vi "Menu Button - Update To Active Level.vi"(7 "RadioButtonsControl in":refnum<vi>, 11 "Display State In in":T1={"Header"="", "Label[]"=[], "DisableButtonsLUT"=variant(string[] []), "Menu Config"=variant}) -> (3 "Display State In out":T1={"Header"="", "Label[]"=[], "DisableButtonsLUT"=variant(string[] []), "Menu Config"=variant})   [LabVIEW 2019, in "Menu Button.xctl"]
doc: "JSMA Module Template - Top Level UI 0.2.0.4\nRob Humfeld - Jet Engineering\nCopyright (c) 2019, Jet Engineering"
uses:
  Menu Button.xctl
  State 1.ctl
  Button Config Cluster STYP.ctl
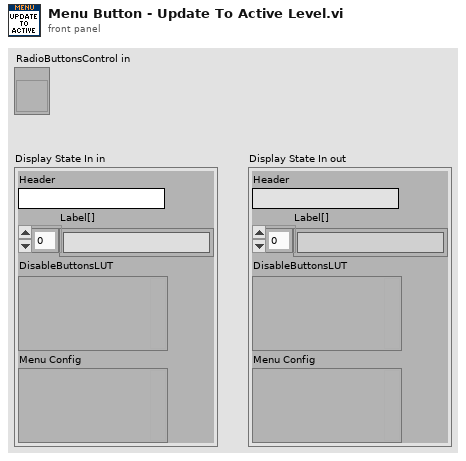
[diagram p1: front panel]
types:
  T1 = typedef "Menu Button.xctl/State 1.ctl" = cluster{"Header":string, "Label[]":string[], "DisableButtonsLUT":variant, "Menu Config":variant}
  T2 = typedef "Menu Button.xctl/Button Config Cluster STYP.ctl" = cluster{"ID":string, "Name":string, "Action":string, "Value":string, "Enable?":bool, "Color":string}
  T3 = typedef "Menu Button.xctl/Level Config Cluster STYP.ctl" = cluster{"ID":string, "Label":string, "Button.ID[]":string[]}
  T4 = enum8{"Enabled", "Disabled", "Disabled and Grayed Out"}
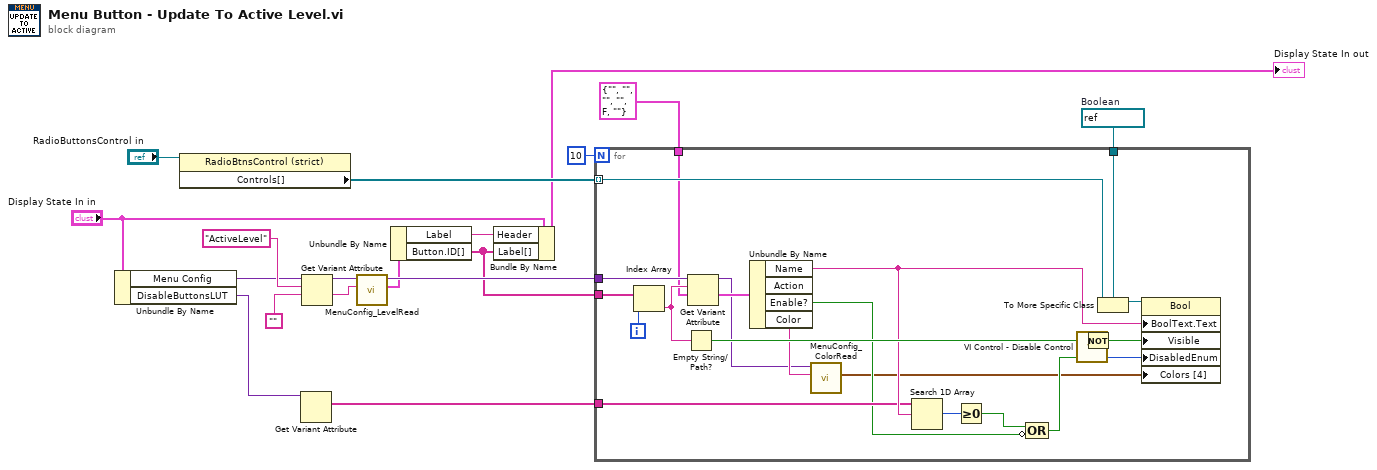
[diagram p0: block diagram]
diagram:
  w18 = refnum<vi> refnum  # Boolean
  n1 = Unbundle By Name("Display State In in") -> ("Menu Config"=w14:variant, "DisableButtonsLUT"=w9:variant)
  n2 = property on="Property Node" class="RadioBtnsControl (strict)"(reference="RadioButtonsControl in") -> ("Controls[]"=w17:refnum<vi>[])  [unwired: 1 in, 2 out]
  n3 = Get Variant Attribute(Variant=w9) -> (names=w8:string[])  [unwired: 3 in, 3 out]
  n4 = Get Variant Attribute(Variant=w14, name="ActiveLevel", default value (empty Variant)="") -> (duplicate Variant=w6:variant, value=w3:string)  [unwired: 1 in, 2 out]
  n5 = call "MenuConfig_LevelRead.vi"("Level.ID"=w3, "MenuConfig"=w6) -> ("LevelConfig"=w4:T3, "MenuConfig"=w5:variant)  [unwired: 7 in, 1 out]
  n6 = Unbundle By Name(w4) -> ("Label"=w2:string, "Button.ID[]"=w1:string[])
  n7 = Bundle By Name(cluster="Display State In in", "Header"=w2, "Label[]"=w1) -> (→"Display State In out":T1)
  n8 = for {
    N: 10 -> [_]
    tunnel: w17 -> [w25] mode=indexing
    tunnel: w18 -> [w38]
    tunnel: w1 -> [w37]
    tunnel: w5 -> [w24]
    tunnel: T2 {"ID"="", "Name"="", "Action"="", "Value"="", "Enable?"=FALSE, "Color"=""} ("ButtonConfig") -> [w23]
    tunnel: w8 -> [w30]
    i -> [w36]
    n9 = Index Array(array=w37, index=w36) -> (element=w34:string)
    n10 = Empty String/Path?(string/path=w34) -> (empty?=w33:bool)
    n11 = Get Variant Attribute(Variant=w24, name=w34, default value (empty Variant)=w23) -> (duplicate Variant=w20:variant, value=w22:T2)  [unwired: 1 in, 2 out]
    n12 = Unbundle By Name(w22) -> ("Name"=w31:string, "Enable?"=w27:bool, "Color"=w21:string)  [unwired: 1 out]
    n13 = call "MenuConfig_ColorRead.vi"("Color.Name (\"Default\")"=w21, "MenuConfig"=w20) -> ("Colors[4]"=w19:cluster{u32, u32}[])  [unwired: 7 in, 2 out]
    n14 = Search 1D Array(1D array=w30, element=w31) -> (index of element=w29:i32)  [unwired: 1 in]
    n15 = Greater Or Equal To 0?(x=w29) -> (x >= 0?=w28:bool)
    n16 = Compound Arithmetic op=OR(w28, invert w27) -> (w26:bool)
    n17 = call <userlib>:"VI Control - Disable Control.vi"("Disable? (T)"=w26) -> ("Disabled Attribute"=w35:T4)  [unwired: 7 in, 1 out]
    n18 = Not(x=w33) -> (.not. x?=w32:bool)
    n19 = To More Specific Class(target class=w38, reference=w25) -> (specific class reference=w39:refnum<vi>)  [unwired: 1 in, 1 out]
    n20 = property class="Bool"(reference=w39, "BoolText.Text"=w31, "Visible"=w32, "DisabledEnum"=w35, "Colors [4]"=w19) -> ()  [unwired: 1 in, 2 out]
  }
